vi "KH7008 Get All Channels.vi"(8 "error in (no error)":errorcluster, 11 "VISA Refnum in":refnum<visa-resource-name>="COM1") -> (0 "error out":errorcluster, 2 "Channel Parameters []":T1[](array[typedef]), 3 "VISA Refnum out":refnum<visa-resource-name>)   [LabVIEW 2019, in "Inst.Krohn-Hite-7008.lvclass"]
uses:
  Inst.Krohn-Hite-7008.lvclass
  Typedefs/Channel-Enum.ctl
  Typedefs/SetAll-Cluster.ctl
  Typedefs/Filter-Enum.ctl
  Typedefs/Shunt-Enum.ctl
  Typedefs/Coupling-Enum.ctl
  Typedefs/Input Configuration-Enum.ctl
  Typedefs/Gain-Enum.ctl
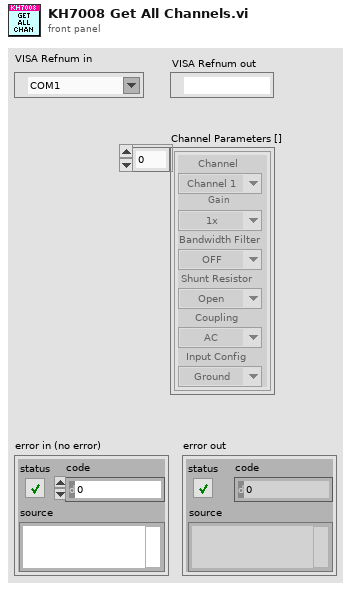
[diagram p1: front panel]
types:
  T1 = typedef "Inst.Krohn-Hite-7008.lvclass/SetAll-Cluster.ctl" = cluster{"Channel":T2, "Gain":T3, "Bandwidth Filter":T4, "Shunt Resistor":T5, "Coupling":T6, "Input Config":T7}
  T2 = typedef "Inst.Krohn-Hite-7008.lvclass/Channel-Enum.ctl" = enum16{"Channel 1", "Channel 2", "Channel 3", "Channel 4", "Channel 5", "Channel 6", "Channel 7", "Channel 8"}
  T3 = typedef "Inst.Krohn-Hite-7008.lvclass/Gain-Enum.ctl" = enum16{"1x", "10x", "100x", "1000x"}
  T4 = typedef "Inst.Krohn-Hite-7008.lvclass/Filter-Enum.ctl" = enum16{"OFF", "ON"}
  T5 = typedef "Inst.Krohn-Hite-7008.lvclass/Shunt-Enum.ctl" = enum16{"Open", "50 Ohms", "500 Ohms", "5k Ohms", "50k Ohms", "10M Ohm"}
  T6 = typedef "Inst.Krohn-Hite-7008.lvclass/Coupling-Enum.ctl" = enum16{"AC", "DC"}
  T7 = typedef "Inst.Krohn-Hite-7008.lvclass/Input Configuration-Enum.ctl" = enum16{"Ground", "SE+ (-gnd)", "SE- (+gnd)", "Differential"}
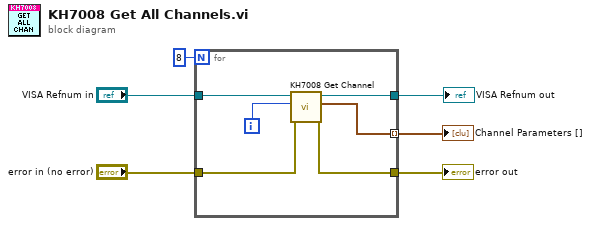
[diagram p0: block diagram]
diagram:
  n1 = for {
    N: 8 -> [_]
    tunnel: "VISA Refnum in" -> [w12]
    tunnel: [w11] -> w5
    tunnel: "error in (no error)" -> [w10]
    tunnel: [w9] -> w3
    tunnel: [w7] -> w2 mode=indexing
    i -> [w8]
    n2 = call "KH7008 Get Channel.vi"("error in (no error)"=w10, "Channel"=w8, "VISA Refnum in"=w12) -> ("error out"=w9:errorcluster, "Channel Parameters"=w7:T1, "VISA Refnum out"=w11:refnum<visa-resource-name>)  [unwired: 6 in]
  }
  "error out" <- w3
  "VISA Refnum out" <- w5
  "Channel Parameters []" <- w2
